vi "relay commands to message handler.vi"(9 "Comms data":T1={"Parameters"={"error writer name"="error writer", "command reader name"="command reader", "error buffer size"=16, "command buffer size"=16, "scanivalveIP"="", "scanivalvePeriod"=16}, "Variables"={"listen schedule"=0, "incident buffer"=[], "command stream"="", "error stream"="", "waiting for command stream connect"=FALSE, "waiting for error stream connect"=FALSE, "scanivalve connection"=refnum, "scanivalveScheduleID"=16}}, 11 "RT Queues":T3) -> ()   [LabVIEW 2018]
uses:
  Type Defs/Queues cluster.ctl
  Chris VIs/Message Scheduler/message scheduler.lvclass
  comms data.ctl
  Type Defs/generic incident.ctl
  Queue VIs/En-queue RT message element.vi
  Chris VIs/Message Scheduler/scheduled message/scheduled message.lvclass
  <resource>/objmgr/ni.dex.rc
types:
  T1 = typedef "comms data.ctl" = cluster{"Parameters":cluster{"error writer name":string, "command reader name":string, "error buffer size":i32, "command buffer size":i32, "scanivalveIP":string, "scanivalvePeriod":u16}, "Variables":cluster{"listen schedule":u32, "incident buffer":T2[], "command stream":refnum<k21>, "error stream":refnum<k21>, "waiting for command stream connect":bool, "waiting for error stream connect":bool, "scanivalve connection":refnum<k5>, "scanivalveScheduleID":u32}}
  T2 = typedef "generic incident.ctl" = cluster{"timestamp":timestamp, "type":string, "Variant":variant}
  T3 = typedef "Queues cluster.ctl" = cluster{"RT Message":refnum<queue>, "RT Comms":refnum<queue>, "RT Data":refnum<queue>, "RT FIFO":refnum<queue>, "message scheduler":refnum<class "message scheduler.lvclass">}
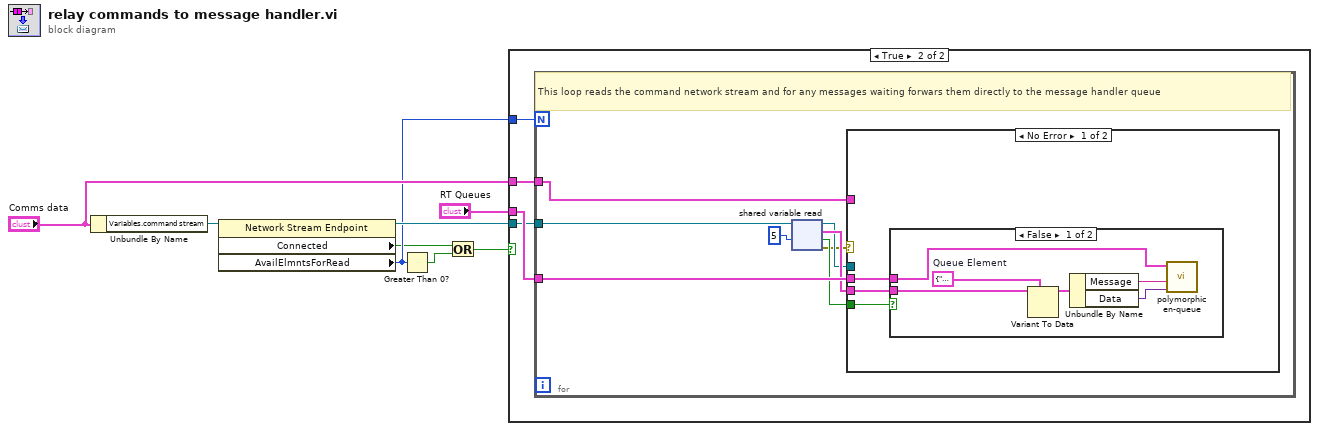
[diagram p0: block diagram]
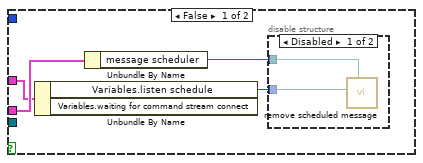
[diagram p2: hidden frame]
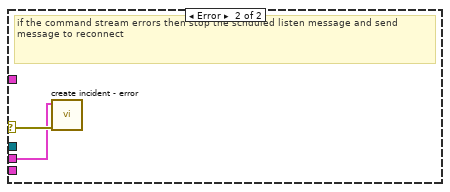
[diagram p5: hidden frame]
diagram:
  n1 = Unbundle By Name("Comms data") -> ("Variables.command stream"=w6:refnum<k21>)
  n2 = property class="Network Stream Endpoint"(reference=w6) -> (reference out=w5:refnum<k21>, "Connected"=w2:bool, "AvailElmntsForRead"=w4:i32)  [unwired: 1 in, 1 out]
  n3 = Greater Than 0?(x=w4) -> (x > 0?=w3:bool)
  n4 = Or(x=w2, y=w3) -> (x .or. y?=w1:bool)
  n5 = case shown="True" w1 {
    tunnel: "RT Queues" -> [w12 w18]
    tunnel: "Comms data" -> [w11 w17]
    tunnel: w5 -> [_ w16]
    tunnel: w4 -> [_ w15]
    frame False {
      n6 = Unbundle By Name(w11) -> ("Variables.listen schedule"=w9:u32)  [unwired: 1 out]
      n7 = Unbundle By Name(w12) -> ("message scheduler"=w10:refnum<class "message scheduler.lvclass">)
      n8 = disable-structure shown="Disabled" {
        disable-tunnel: w10 -> [w14 _]
        disable-tunnel: w9 -> [w13 _]
        frame Disabled {
          n9 = call "remove scheduled message.vi"("message scheduler"=w14, "schedule ID"=w13) -> ()  [unwired: 9 in, 1 out]
        }
        frame Enabled {
        }
      }
    }
    frame True {
      n10 = for {
        N: w15 -> [_]
        tunnel: w16 -> [w26]
        tunnel: w18 -> [w24]
        tunnel: w17 -> [w22]
        # "This loop reads the command network stream and for any messages waiting forwars them directly to the message handler queue"
        n11 = shared-variable-read(w26, 5 ("timeout ms (-1)")) -> (w21:refnum<k21>, w19:errorcluster, w20:bool, w23:cluster{"message":string, "data":variant})  [unwired: 1 in]
        n12 = case shown="No Error" w19 {
          selector: w19 -> [_ w37]
          tunnel: w24 -> [w29 w36]
          tunnel: w23 -> [w28 _]
          tunnel: w20 -> [w27 _]
          tunnel: w22 -> [_ _]
          tunnel: w21 -> [_ _]
          frame No Error {
            n13 = case shown="False" w27 {
              tunnel: w29 -> [w35 _]
              tunnel: w28 -> [w34 _]
              frame False {
                w30 = cluster{"Message":string, "Data":variant} {"Message"="", "Data"=variant}  # Queue Element
                n14 = Variant To Data(type=w30, Variant=w34) -> (data=w33:cluster{"Message":string, "Data":variant})  [unwired: 1 in, 1 out]
                n15 = Unbundle By Name(w33) -> ("Message"=w32:string, "Data"=w31:variant)
                n16 = call-poly "polymorphic en-queue.vi"("Data"=w31, "Message"=w32, "RT Queues"=w35) -> ()  [unwired: 8 in, 1 out]
              }
              frame True {
              }
            }
          }
          frame Error {
            # "if the command stream errors then stop the schduled listen message and send message to reconnect"
            n17 = call "create incident - error.vi"("error"=w37, "RT Queues"=w36) -> ()  [unwired: 9 in, 1 out]
          }
        }
      }
    }
  }
